vi "viewAndTarget.vi"() -> ()   [LabVIEW 2017]
uses:
  globalUtilities.vi
  <vilib>/Utility/file.llb/Write Delimited Spreadsheet (I64).vi
  globalDevices.vi
  getComputerName.vi
panel:
  out "el time":dbl
  out "folder name":string
  in  "framesSave":bool
  in  "target":bool=TRUE
  in  "stop 2":bool
  in  "piezo2 2":dbl=100.0
  in  "open shutter 2":bool
  in  "close shutter 2":bool
  in  "piezo1 2":dbl=100.0 format="%#_13g"
  in  "piezo1":dbl=100.0 format="%03.1f"
  in  "close shutter":bool
  in  "open shutter":bool
  in  "piezo2":dbl=100.0
  in  "stop":bool
  in  "frames per second":dbl=20.0
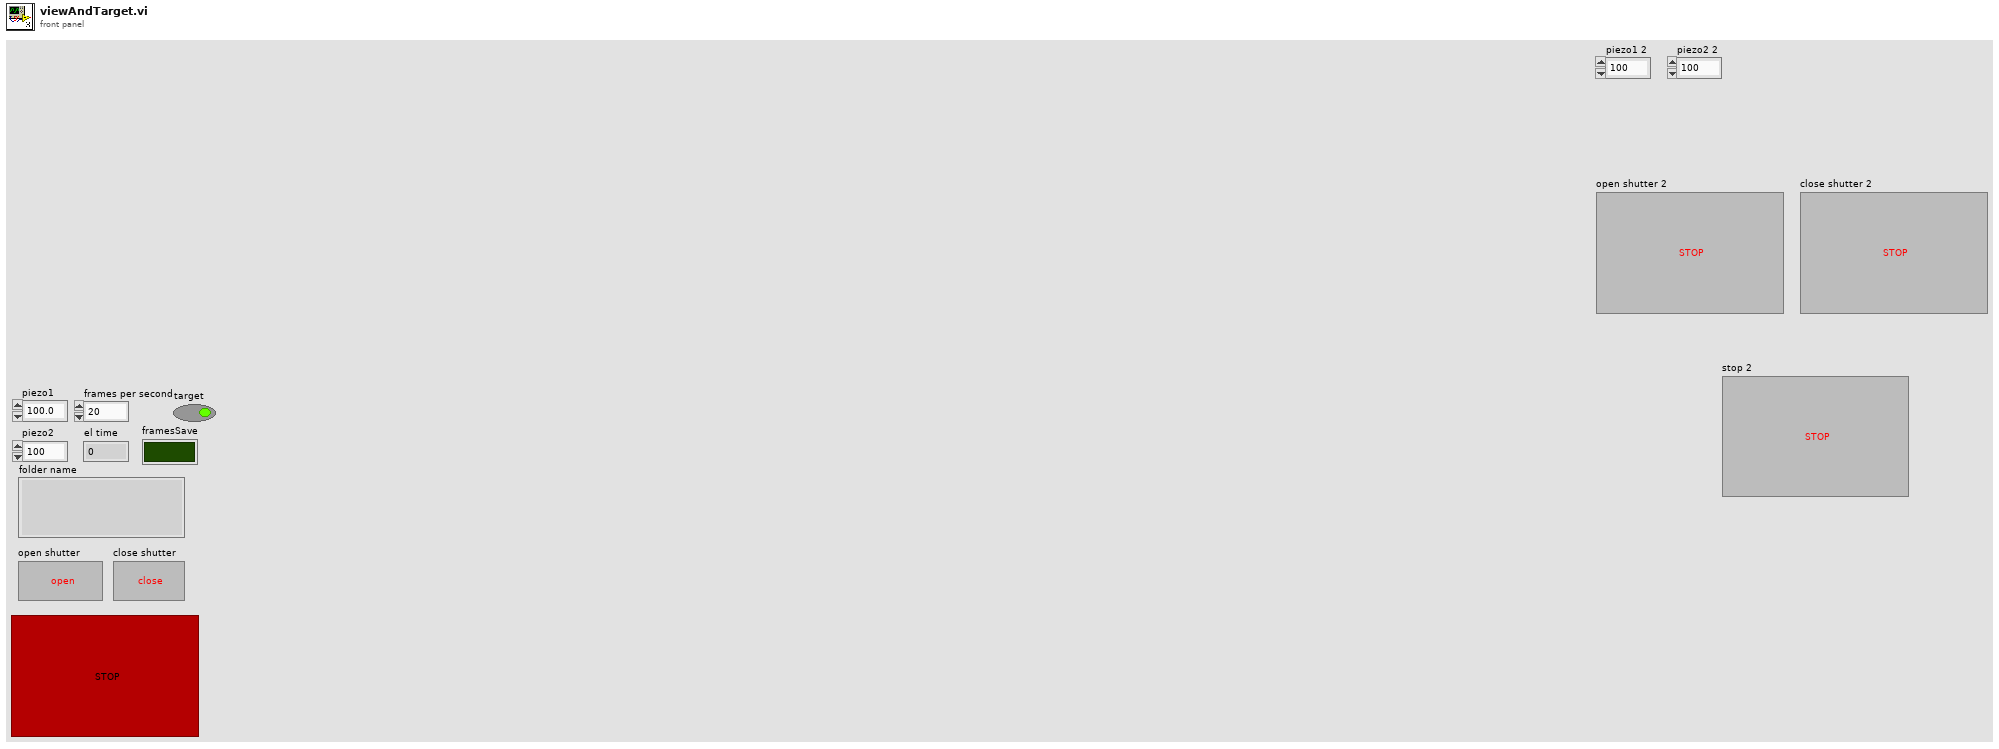
[diagram p1: front panel]
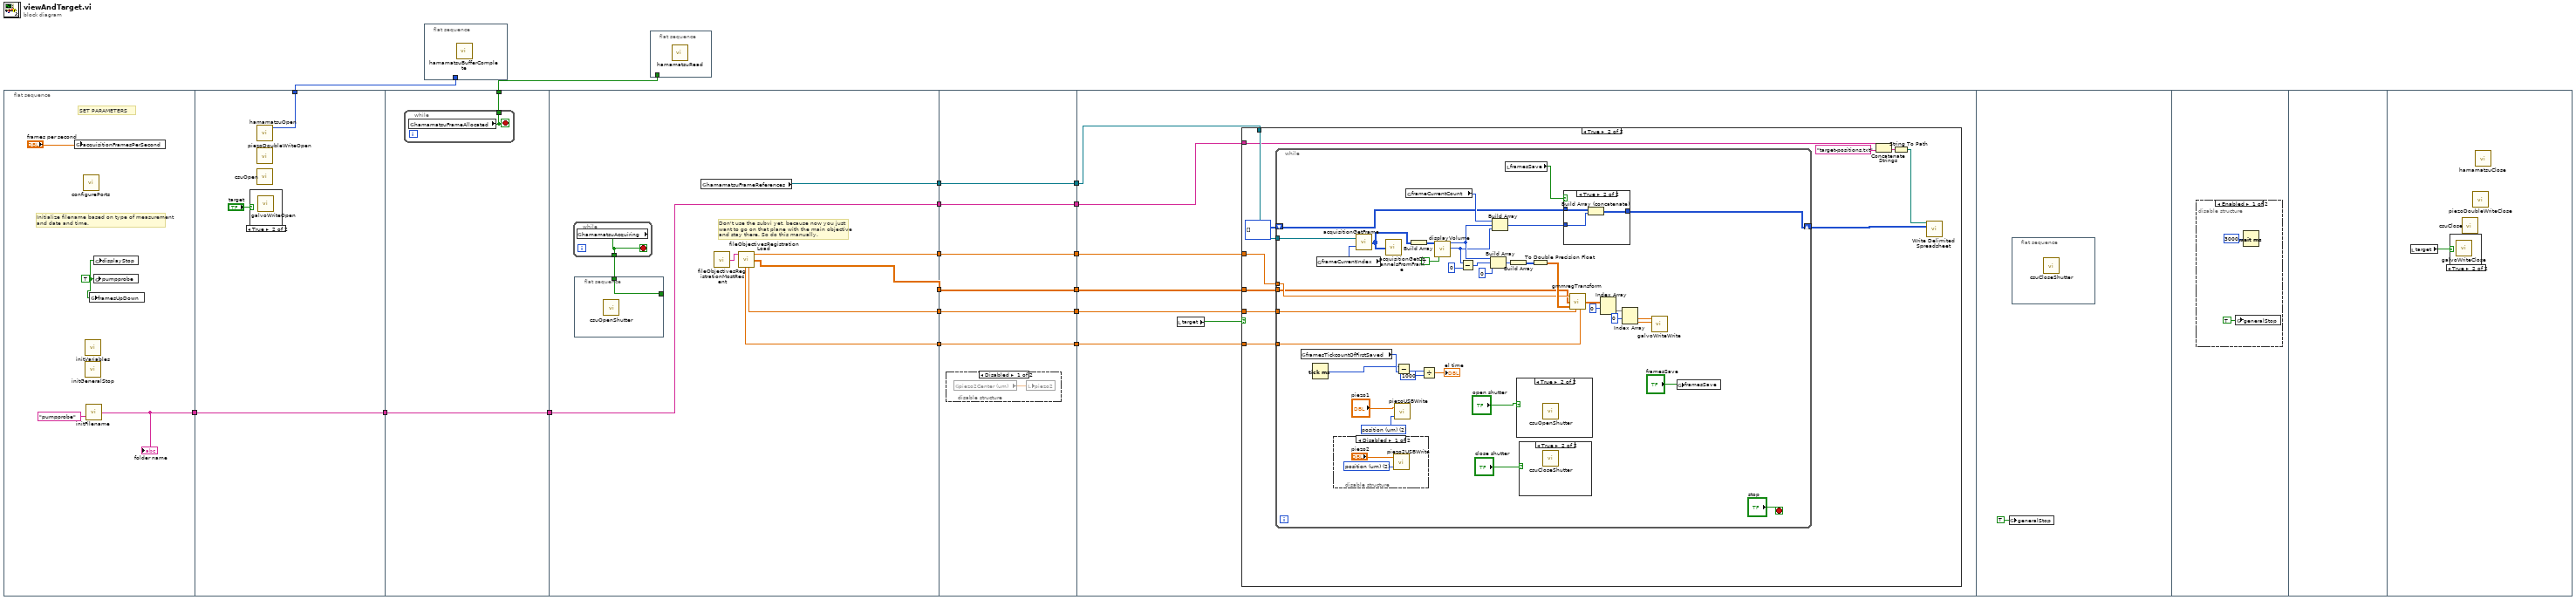
[diagram p0: block diagram]
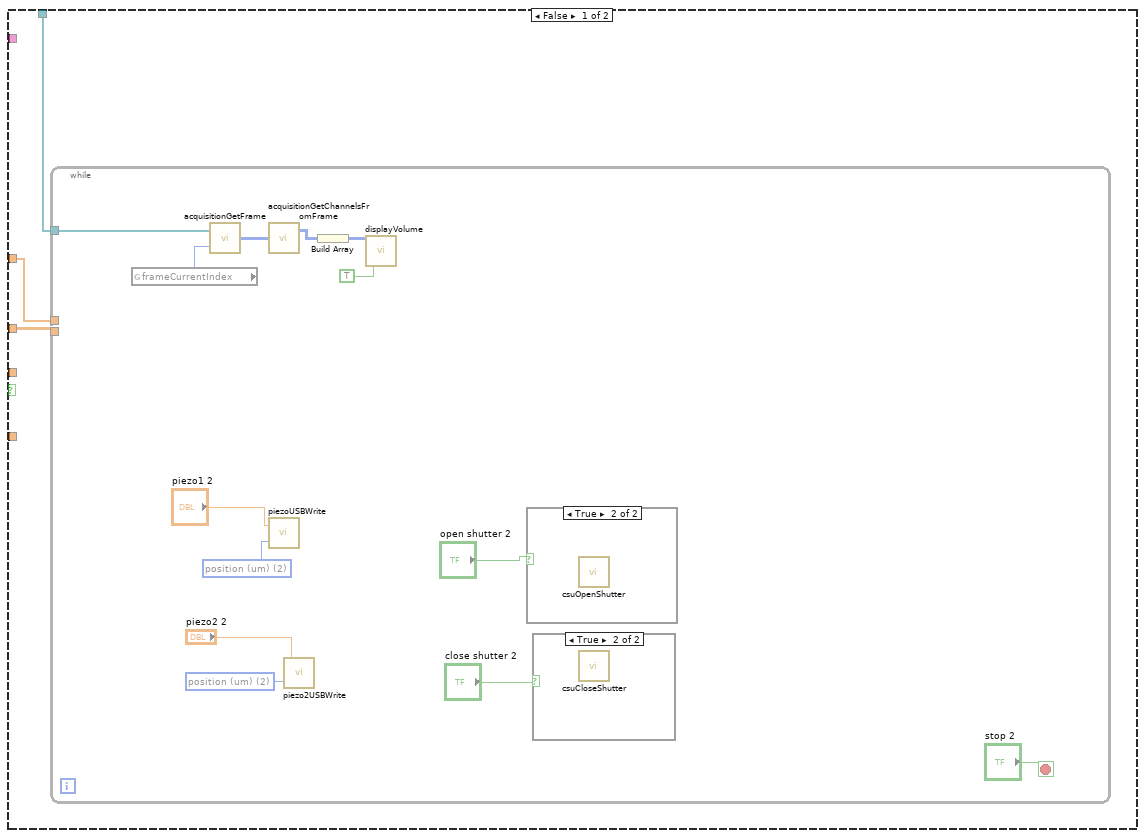
[diagram p4: hidden frame]
diagram:
  n1 = flat-sequence {
    tunnel: [w19] -> w15
    tunnel: [w24] -> w17
    tunnel: [w23] -> w16
    tunnel: w15 -> [w23]
    tunnel: w16 -> [w25]
    tunnel: [w26] -> w14
    tunnel: [w25] -> w2
    tunnel: [w33] -> w13
    tunnel: [w32] -> w11
    tunnel: [w31] -> w9
    tunnel: [w30] -> w7
    tunnel: [w29] -> w5
    tunnel: [w28] -> w3
    tunnel: w2 -> [w28]
    tunnel: w13 -> [w43]
    tunnel: [w43] -> w12
    tunnel: w11 -> [w42]
    tunnel: [w42] -> w10
    tunnel: w9 -> [w41]
    tunnel: [w41] -> w8
    tunnel: w7 -> [w40]
    tunnel: [w40] -> w6
    tunnel: w5 -> [w39]
    tunnel: [w39] -> w4
    tunnel: w3 -> [w38]
    tunnel: [w38] -> w1
    tunnel: w12 -> [w51]
    tunnel: w10 -> [w50]
    tunnel: w8 -> [w49]
    tunnel: w6 -> [w48]
    tunnel: w4 -> [w47]
    tunnel: w1 -> [w45]
    frame #0 {
      w18 = TRUE ("pumpprobe")
      # "SET PARAMETERS"
      # "Initialize filename based on type of measurement\nand date and time."
      n2 = global write "globalUtilities.vi" "acquisitionFramesPerSecond"("frames per second") -> ()
      n3 = call "configurePorts.vi"() -> ()  [unwired: 12 in]
      n4 = call "initVariables.vi"() -> ()  [unwired: 12 in]
      n5 = call "initGeneralStop.vi"() -> ()  [unwired: 1 in]
      n6 = call "initFilename.vi"("Experiment type"="pumpprobe") -> ("folder name"=w19:string)  [unwired: 1 in]
      "folder name" <- w19
      n7 = global write "globalUtilities.vi" "framesUpDown"(w18) -> ()
      n8 = global write "globalUtilities.vi" "pumpprobe"(w18) -> ()
      n9 = global write "globalUtilities.vi" "displayStop"(w18) -> ()
    }
    frame #1 {
      n10 = case shown="True" "target" {
        frame False {
        }
        frame True {
          n11 = call "galvoWriteOpen.vi"() -> ()  [unwired: 12 in]
        }
      }
      n12 = call "hamamatsuOpen.vi"() -> ("Handle out"=w24:u32)  [unwired: 3 out]
      n13 = call "piezoDoubleWriteOpen.vi"() -> ()  [unwired: 2 in]
      n14 = call "csuOpen.vi"() -> ()  [unwired: 14 in, 2 out]
    }
    frame #2 {
      n15 = while {
        tunnel: [w27] -> w26
        stop <- w27 stop-if-true
        n16 = global read "globalDevices.vi" "hamamatsuFrameAllocated"() -> (w27:bool)
      }
    }
    frame #3 {
      # "Don't use the subvi yet, because now you just\nwant to go on that plane with the main objective\nand stay there. So do this manually."
      n17 = while {
        tunnel: [w37] -> w35
        stop <- w37 stop-if-true
        n18 = global read "globalUtilities.vi" "hamamatsuAcquiring"() -> (w37:bool)
      }
      n19 = flat-sequence {
        tunnel: w35 -> [w36]
        tunnel: [w36] -> _
        frame #0 {
          n20 = call "csuOpenShutter.vi"() -> ()  [unwired: 16 in]
        }
      }
      n21 = global read "globalDevices.vi" "hamamatsuFrameReferences"() -> (w33:refnum<data-value>[])
      n22 = call "fileObjectivesRegistrationMostRecent.vi"() -> ("f"=w34:string)  [unwired: 1 in]
      n23 = call "fileObjectivesRegistrationLoad.vi"("objectiveRegistrationFilePath"=w34) -> ("denormParam"=w29:dbl[], "param"=w32:dbl[], "imaging (model)"=w31:dbl[][], "normParam"=w30:dbl[])  [unwired: 3 in, 2 out]
    }
    frame #4 {
      n24 = disable-structure shown="Disabled" {
        frame Disabled {
          n25 = global read "globalDevices.vi" "piezo2Center (um)"() -> (w44:dbl)
          n26 = local write "piezo2"(w44) -> ()
        }
        frame Enabled {
        }
      }
    }
    frame #5 {
      n27 = local read "target"() -> (w46:bool)
      n28 = case shown="True" w46 {
        tunnel: w51 -> [w52 w78]
        tunnel: w50 -> [w54 w77]
        tunnel: w49 -> [w53 w76]
        tunnel: w48 -> [_ w75]
        tunnel: w47 -> [_ w74]
        tunnel: w45 -> [_ w72]
        frame False {
          n29 = while {
            tunnel: w52 -> [w65]
            tunnel: w54 -> [_]
            tunnel: w53 -> [_]
            stop <- "stop 2" stop-if-true
            w60 = u16 2 items=["fractional", "voltage (V)", "position (um)"] ("mode")
            w62 = u16 2 items=["fractional", "voltage (V)", "position (um)"] ("mode")
            n30 = global read "globalUtilities.vi" "frameCurrentIndex"() -> (w66:i32)
            n31 = call "acquisitionGetFrame.vi"("index"=w66, "hamamatsuFrameReferences"=w65) -> ("frameOut"=w56:u16[][])
            n32 = call "acquisitionGetChannelsFromFrame.vi"("frameIn"=w56) -> ("Red"=w55:u16[][])  [unwired: 1 out]
            n33 = call "piezoUSBWrite.vi"("mode"=w62, "position"="piezo1 2") -> ()  [unwired: 1 in]
            n34 = call "piezo2USBWrite.vi"("mode"=w60, "position"="piezo2 2") -> ()  [unwired: 1 in]
            n35 = Build Array(w55) -> (w64:u16[][][])
            n36 = call "displayVolume.vi"("frames"=w64, "stop immediately"=TRUE) -> ()  [unwired: 12 in, 6 out]
            n37 = case shown="True" "open shutter 2" {
              frame False {
              }
              frame True {
                n38 = call "csuOpenShutter.vi"() -> ()  [unwired: 16 in]
              }
            }
            n39 = case shown="True" "close shutter 2" {
              frame False {
              }
              frame True {
                n40 = call "csuCloseShutter.vi"() -> ()  [unwired: 16 in]
              }
            }
          }
        }
        frame True {
          n41 = while {
            tunnel: w78 -> [w115]
            tunnel: w77 -> [w103]
            tunnel: w76 -> [w102]
            tunnel: w75 -> [w96]
            tunnel: w74 -> [w95]
            shift-right: [w85] -> w73
            shift-left: i32[][] [] -> [w86]
            stop <- "stop" stop-if-true
            w100 = u16 2 items=["fractional", "voltage (V)", "position (um)"] ("mode")
            n42 = global read "globalUtilities.vi" "framesTickcountOfFirstSaved"() -> (w80:u32)
            n43 = Tick Count (ms)() -> (millisecond timer value=w79:u32)
            n44 = global read "globalUtilities.vi" "frameCurrentIndex"() -> (w116:i32)
            n45 = disable-structure shown="Disabled" {
              frame Disabled {
                w118 = u16 2 items=["fractional", "voltage (V)", "position (um)"] ("mode")
                n46 = call "piezo2USBWrite.vi"("mode"=w118, "position"="piezo2") -> ()  [unwired: 1 in]
              }
              frame Enabled {
              }
            }
            n47 = call "acquisitionGetFrame.vi"("index"=w116, "hamamatsuFrameReferences"=w115) -> ("frameOut"=w94:u16[][])
            n48 = call "acquisitionGetChannelsFromFrame.vi"("frameIn"=w94) -> ()  [unwired: 2 out]
            n49 = call "piezoUSBWrite.vi"("mode"=w100, "position"="piezo1") -> ()  [unwired: 1 in]
            n50 = Subtract(x=w79, y=w80) -> (x-y=w83:u32)
            n51 = global read "globalUtilities.vi" "frameCurrentCount"() -> (w88:i32)
            n52 = Build Array(w94) -> (w114:u16[][][])
            n53 = Divide(x=w83, y=u32 1000) -> (x/y=→"el time":dbl)
            n54 = call "displayVolume.vi"("frames"=w114, "stop immediately"=TRUE) -> ("X0out"=w90:i32, "Y0out"=w89:i32)  [unwired: 12 in, 4 out]
            n55 = Subtract(x=w89, y=0) -> (x-y=w92:i32)
            n56 = Build Array(w90, w92, 0 ("element")) -> (w105:i32[])
            n57 = Build Array(w88, w90, w89) -> (w87:i32[])
            n58 = local read "framesSave"() -> (w84:bool)
            n59 = Build Array(w105) -> (w106:i32[][])
            n60 = case shown="True" "open shutter" {
              frame False {
              }
              frame True {
                n61 = call "csuOpenShutter.vi"() -> ()  [unwired: 16 in]
              }
            }
            n62 = case shown="True" "close shutter" {
              frame False {
              }
              frame True {
                n63 = call "csuCloseShutter.vi"() -> ()  [unwired: 16 in]
              }
            }
            n64 = To Double Precision Float(number=w106) -> (double precision float=w107:dbl[][])
            n65 = case shown="True" w84 {
              tunnel: w87 -> [_ w123]
              tunnel: w86 -> [w120 w122]
              tunnel: [w120 w121] -> w85
              frame False {
              }
              frame True {
                n66 = Build Array (concatenate)(w122, w123) -> (w121:i32[][])
              }
            }
            n67 = call "gmmregTransform.vi"("param0"=w103, "ctrlPts"=w102, "pts"=w107, "normParams"=w96, "denormParams"=w95) -> ("out"=w108:dbl[][])  [unwired: 4 in]
            n68 = Index Array(array=w108, index (row)=0) -> (element=w110:dbl[])  [unwired: 1 in]
            n69 = Index Array(array=w110, index #1=0 ("index")) -> (element #1=w112:dbl, element #2=w113:dbl)  [unwired: 1 in]
            n70 = call "galvoWriteWrite.vi"("X"=w112, "Y"=w113) -> ()  [unwired: 4 in]
            n71 = global write "globalUtilities.vi" "framesSave"("framesSave") -> ()
          }
          n72 = Concatenate Strings(w72, "target-positions.txt" ("string")) -> (w70:string)
          n73 = String To Path(string=w70) -> (path=w69:path)
          n74 = call-poly <vilib>:"Write Delimited Spreadsheet.vi"("file path (dialog if empty)"=w69, "2D data"=w73) -> ()  [unwired: 12 in, 2 out]
        }
      }
    }
    frame #6 {
      n75 = global write "globalUtilities.vi" "generalStop"(TRUE ("generalStop")) -> ()
      n76 = flat-sequence {
        frame #0 {
          n77 = call "csuCloseShutter.vi"() -> ()  [unwired: 16 in]
        }
      }
    }
    frame #7 {
      n78 = disable-structure shown="Enabled" {
        frame Enabled {
          n79 = global write "globalUtilities.vi" "generalStop"(TRUE ("generalStop")) -> ()
          n80 = Wait (ms)(milliseconds to wait=u32 3000) -> ()  [unwired: 1 out]
        }
        frame Disabled {
        }
      }
    }
    frame #8 {
    }
    frame #9 {
      n81 = local read "target"() -> (w127:bool)
      n82 = case shown="True" w127 {
        frame False {
        }
        frame True {
          n83 = call "galvoWriteClose.vi"() -> ()  [unwired: 12 in]
        }
      }
      n84 = call "csuClose.vi"() -> ()  [unwired: 12 in]
      n85 = call "piezoDoubleWriteClose.vi"() -> ()  [unwired: 1 in]
      n86 = call "hamamatsuClose.vi"() -> ()  [unwired: 1 out]
    }
  }
  n87 = flat-sequence {
    tunnel: w17 -> [_]
    frame #0 {
      n88 = call "hamamatsuBufferComplete.vi"() -> ()  [unwired: 12 in]
    }
  }
  n89 = flat-sequence {
    tunnel: w14 -> [_]
    frame #0 {
      n90 = call "hamamatsuRead.vi"() -> ()  [unwired: 12 in]
    }
  }
